vi "check_any_corner_islands.vi"(2 "tour_in_progress":T1[](array[typedef]), 3 "chessboard":T2[][](array[typedef])) -> (0 "corner square that starts an island":T1, 1 "T = a corner island was found":bool)   [LabVIEW 2020, in "core.lvlib"]
doc: "This VI outputs TRUE if one or more \"corner islands\" were found.\nAn \"island\" is a group of unreacheable squares. A \"corner island\" is an island that has one end in the corner. \n\nA corner island could be the squares \"a8-b6-c4\" (if all their neighbouring squares are explored, and none of them are the head of the tour (the current square))."
uses:
  core.lvlib
  core_data/chessboard_index.ctl
  core_data/chess_square.ctl
  core_data/neighbour_square.ctl
  check_head_is_neighbour.vi
  get_chessboard_square.vi
  get all unexplored neighbours.vi
  core_data/core_data.lvlib
  core_data/file--enum.ctl
  core_data/rank--enum.ctl
  core_data/chess_square--chess notation.ctl
panel:
  # "Development\ncontrols/indicators useful for development and testing, but which are not outputs of the VI"
  # "Input\nInputs to the VI"
  # "Output\nOutputs of the VI"
  # "Description\n\nBlank VI with error handling case. \n\nSummarize the use of this VI in this space."
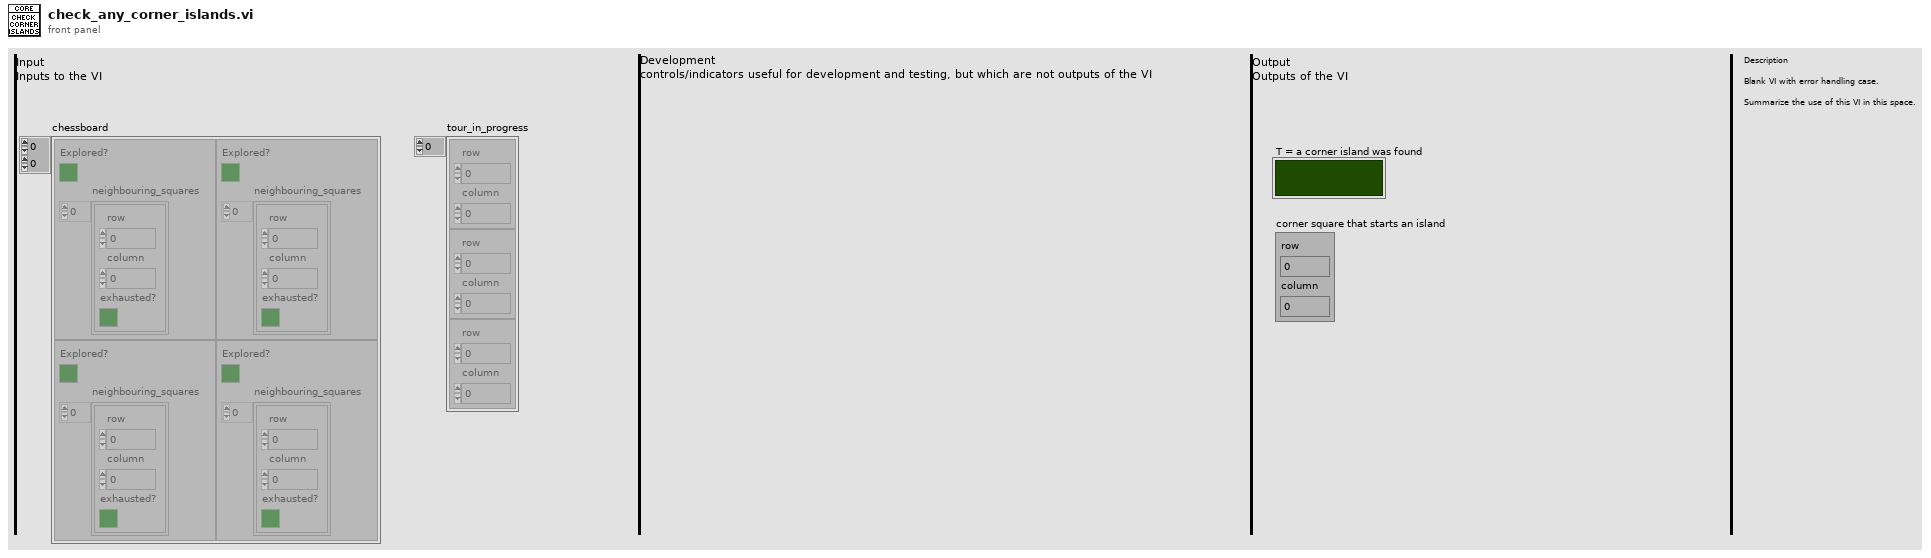
[diagram p1: front panel]
types:
  T1 = typedef "core.lvlib/core_data.lvlib/chessboard_index.ctl" = cluster{"row":u8, "column":u8}
  T2 = typedef "core.lvlib/core_data.lvlib/chess_square.ctl" = cluster{"Explored?":bool, "neighbouring_squares":T3[]}
  T3 = typedef "core.lvlib/core_data.lvlib/neighbour_square.ctl" = cluster{"row":u8, "column":u8, "exhausted?":bool}
  T4 = typedef "core.lvlib/core_data.lvlib/chess_square--chess notation.ctl" = cluster{"file":T5, "rank":T6}
  T5 = typedef "core.lvlib/core_data.lvlib/file--enum.ctl" = enum16{"a", "b", "c", "d", "e", "f", "g", "h"}
  T6 = typedef "core.lvlib/core_data.lvlib/rank--enum.ctl" = enum16{"1", "2", "3", "4", "5", "6", "7", "8"}
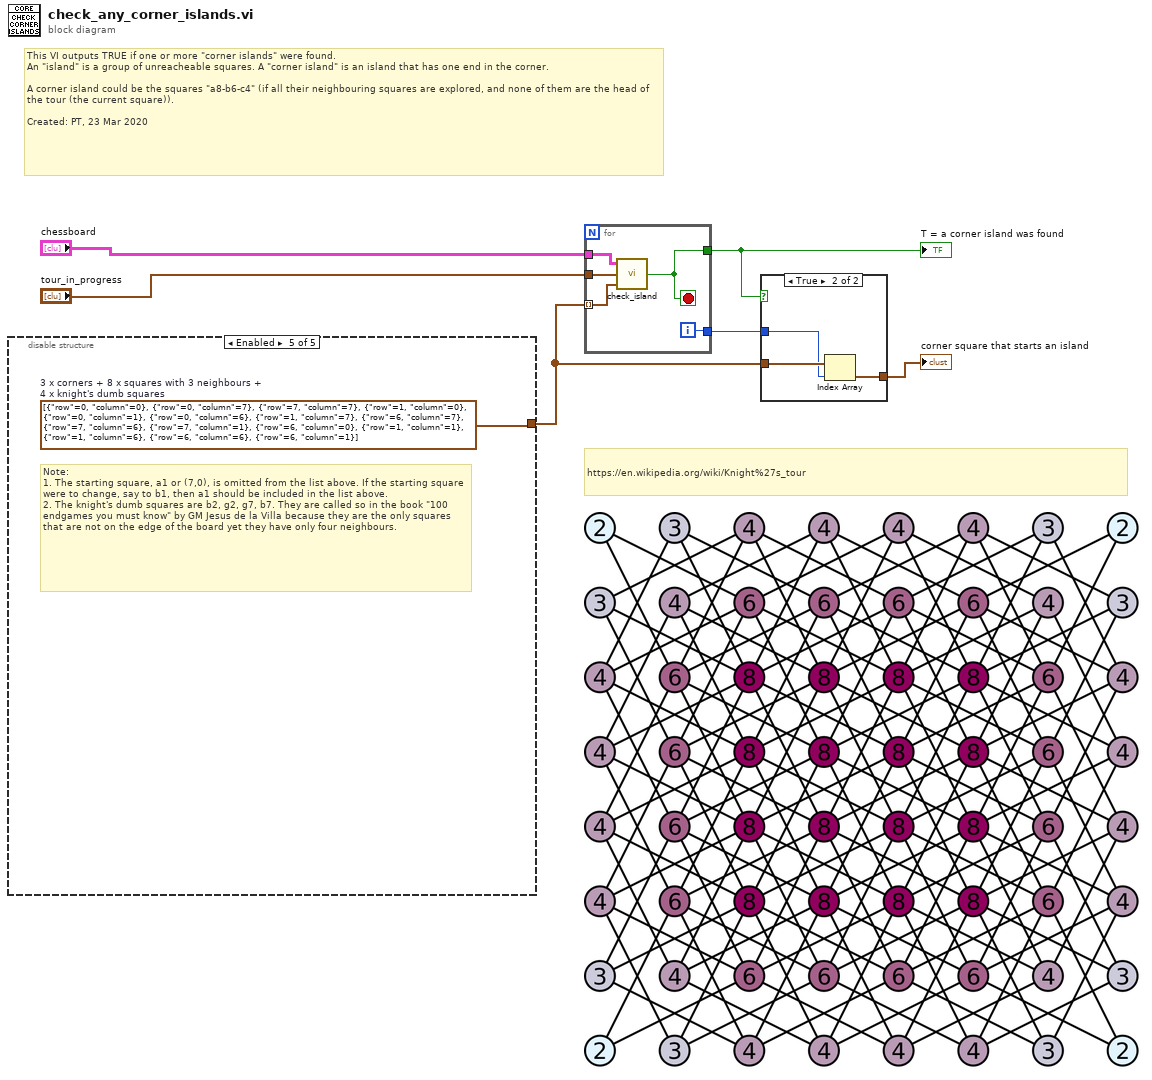
[diagram p0: block diagram]
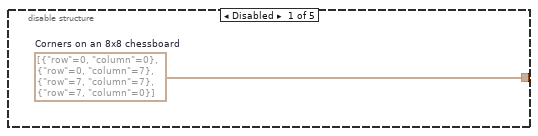
[diagram p2: hidden frame]
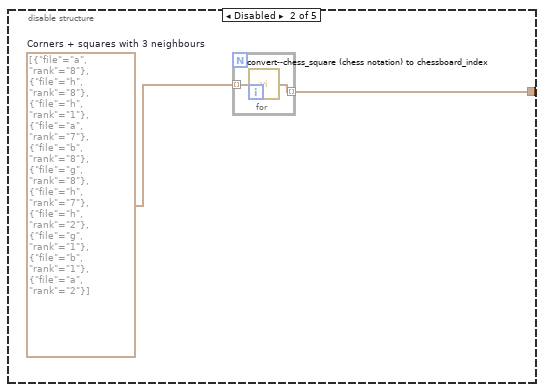
[diagram p3: hidden frame]
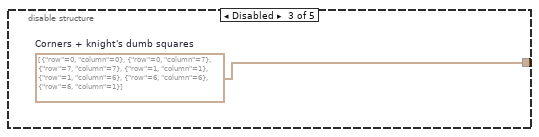
[diagram p4: hidden frame]
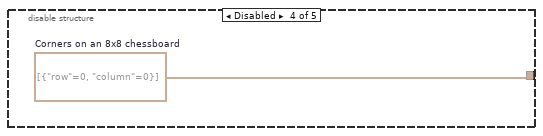
[diagram p5: hidden frame]
diagram:
  # "https://en.wikipedia.org/wiki/Knight%27s_tour"
  # "This VI outputs TRUE if one or more \"corner islands\" were found.\nAn \"island\" is a group of unreacheable squares. A \"corner island\" is an island that has one end in the corner. \n\nA corner island could be the squares \"a8-b6-c4\" (if all their neighbouring squares are explored, and none of them are the head of the tour (the current square)).\n\nCreated: PT, 23 Mar 2020"
  n1 = disable-structure shown="Enabled" {
    disable-tunnel: [w7 w9 w12 w13 w14] -> w4
    frame Disabled {
      w7 = T1[] [{"row"=0, "column"=0}, {"row"=0, "column"=7}, {"row"=7, "column"=7}, {"row"=7, "column"=0}]  # Corners on an 8x8 chessboard
    }
    frame Disabled {
      w8 = T4[] [{"file"=enum."a", "rank"=enum."8"}, {"file"=enum."h", "rank"=enum."8"}, {"file"=enum."h", "rank"=enum."1"}, {"file"=enum."a", "rank"=enum."7"}, {"file"=enum."b", "rank"=enum."8"}, {"file"=enum."g", "rank"=enum."8"}, {"file"=enum."h", "rank"=enum."7"}, {"file"=enum."h", "rank"=enum."2"}, {"file"=enum."g", "rank"=enum."1"}, {"file"=enum."b", "rank"=enum."1"}, {"file"=enum."a", "rank"=enum."2"}]  # Corners + squares with 3 neighbours
      n2 = for {
        tunnel: [w11] -> w9 mode=indexing
        tunnel: w8 -> [w10] mode=indexing
        n3 = call "convert--chess_square (chess notation) to chessboard_index.vi"("chess_square (chess notation)"=w10) -> ("chessboard_index"=w11:T1)
      }
    }
    frame Disabled {
      w12 = T1[] [{"row"=0, "column"=0}, {"row"=0, "column"=7}, {"row"=7, "column"=7}, {"row"=1, "column"=1}, {"row"=1, "column"=6}, {"row"=6, "column"=6}, {"row"=6, "column"=1}]  # Corners + knight's dumb squares
    }
    frame Disabled {
      w13 = T1[] [{"row"=0, "column"=0}]  # Corners on an 8x8 chessboard
    }
    frame Enabled {
      w14 = T1[] [{"row"=0, "column"=0}, {"row"=0, "column"=7}, {"row"=7, "column"=7}, {"row"=1, "column"=0}, {"row"=0, "column"=1}, {"row"=0, "column"=6}, {"row"=1, "column"=7}, {"row"=6, "column"=7}, {"row"=7, "column"=6}, {"row"=7, "column"=1}, {"row"=6, "column"=0}, {"row"=1, "column"=1}, {"row"=1, "column"=6}, {"row"=6, "column"=6}, {"row"=6, "column"=1}]  # 3 x corners + 8 x squares with 3 neighbours + 4 x knight's dumb squares
      # "Note:\n1. The starting square, a1 or (7,0), is omitted from the list above. If the starting square were to change, say to b1, then a1 should be included in the list above.\n2. The knight's dumb squares are b2, g2, g7, b7. They are called so in the book \"100 endgames you must know\" by GM Jesus de la Villa because they are the only squares that are not on the edge of the board yet they have only four neighbours."
    }
  }
  n4 = for {
    tunnel: w4 -> [w19] mode=indexing
    tunnel: [w18] -> w6
    tunnel: [w17] -> w3
    tunnel: "chessboard" -> [w16]
    tunnel: "tour_in_progress" -> [w15]
    i -> [w17]
    stop <- w18 stop-if-true
    n5 = call "check_island.vi"("start_square"=w19, "tour_in_progress"=w15, "chessboard"=w16) -> ("T = an island was found"=w18:bool)
  }
  "T = a corner island was found" <- w6
  n6 = case shown="True" w6 {
    tunnel: w4 -> [_ w22]
    tunnel: w3 -> [_ w21]
    tunnel: [_ w20] -> w5
    frame False {
    }
    frame True {
      n7 = Index Array(array=w22, index=w21) -> (element=w20:T1)
    }
  }
  "corner square that starts an island" <- w5
